vi "user process.vi"(8 "error in":errorcluster, 11 "Parameters to process":T2) -> (0 "error out":errorcluster, 3 "Results from processing":T1)   [LabVIEW 2013, in "Custom Controller Module runtime.lvclass"]
uses:
  Custom Controller Module runtime.lvclass
  parameter user data.ctl
  result user data.ctl
  <vilib>/addons/control/pid/pid.llb/PID (DBL).vi
  <vilib>/addons/control/pid/NI_PID_pid.lvlib
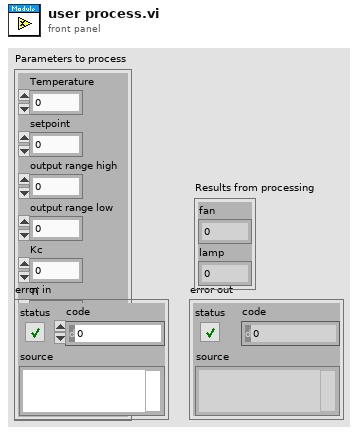
[diagram p1: front panel]
types:
  T1 = typedef "Custom Controller Module runtime.lvclass/result user data.ctl" = cluster{"fan":dbl, "lamp":dbl}
  T2 = typedef "Custom Controller Module runtime.lvclass/parameter user data.ctl" = cluster{"Temperature":dbl, "setpoint":dbl, "output range high":dbl, "output range low":dbl, "Kc":dbl, "Ti":dbl, "Td":dbl, "Fan on?":bool}
  T3 = cluster{"output range high":dbl, "output range low":dbl}
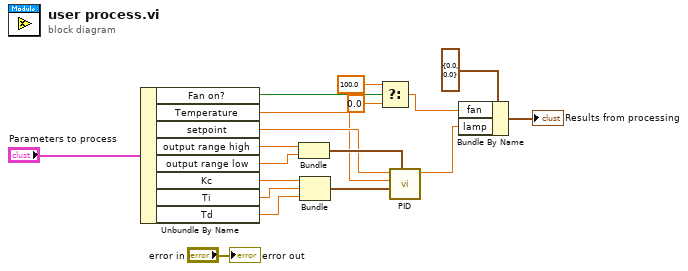
[diagram p0: block diagram]
diagram:
  n1 = Unbundle By Name("Parameters to process") -> ("Fan on?"=w6:bool, "Temperature"=w8:dbl, "setpoint"=w9:dbl, "output range high"=w13:dbl, "output range low"=w12:dbl, "Kc"=w16:dbl, "Ti"=w15:dbl, "Td"=w14:dbl)
  n2 = Bundle("output range high"=w13, "output range low"=w12) -> (w11:T3)  [unwired: 1 in]
  n3 = Bundle("Kc"=w16, "Ti"=w15, "Td"=w14) -> (w10:cluster{"Kc":dbl, "Ti":dbl, "Td":dbl})  [unwired: 1 in]
  n4 = Select(t=100.0, s=w6, f=0.0) -> (s? t:f=w3:dbl)
  n5 = call-poly <vilib>:"PID.vi"("output range"=w11, "PID gains"=w10, "process variable"=w8, "setpoint"=w9) -> ("output"=w2:dbl)  [unwired: 6 in, 1 out]
  n6 = Bundle By Name(cluster=T1 {"fan"=0.0, "lamp"=0.0} ("Results from processing"), "fan"=w3, "lamp"=w2) -> (→"Results from processing":T1)
  "error out" <- "error in"
